vi "获取采配水运行状态.vi"(8 "error in (no error)":errorcluster) -> (0 "error out":errorcluster, 3 "运行流程":T1(ring))   [LabVIEW 2016, in "质控单元V4.lvlib"]
uses:
  <vilib>/Plasmionique/MB Master/MB Master.lvlib
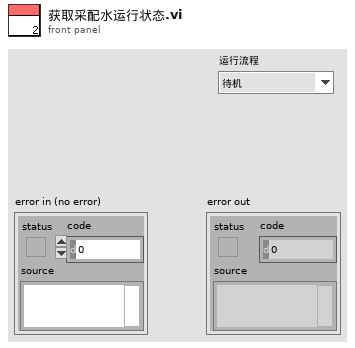
[diagram p1: front panel]
types:
  T1 = enum16{"待机", "初始化", "水样润洗", "一级进水样", "二级进水样", "沉淀", "氨氮水样池进样", "配水", "反冲洗", "储水", "结束"}
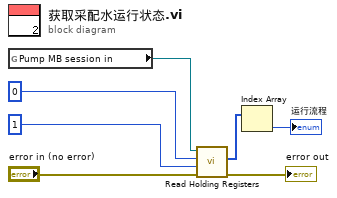
[diagram p0: block diagram]
diagram:
  n1 = global read "系统交互.vi" "Pump MB session in"() -> (w5:refnum<class "MB_Master.lvclass">)
  n2 = call <vilib>:"Read Holding Registers.vi"("error in (no error)"="error in (no error)", "quantity"=u16 1, "starting address"=u16 0, "MB session in"=w5) -> ("error out"=→"error out":errorcluster, "Registers"=w2:u16[])  [unwired: 5 in, 1 out]
  n3 = Index Array(array=w2) -> (element=→"运行流程":u16)  [unwired: 1 in]
